vi "Finish.vi"   [LabVIEW 2012]
doc: "This VI is called just before exiting. It is expected to close I/O refnum, save collected data, etc."
uses:
  <vilib>/Rock Robotics/WPI/Compressor/WPI_CompressorGetSetRefNum.vi
  <vilib>/Rock Robotics/WPI/Joystick/WPI_JoystickGetSetRefNum.vi
  <vilib>/Rock Robotics/WPI/RobotDrive/WPI_RobotDriveGetSetRefNum.vi
types:
  T1 = typedef "WPI_MotorControlDeviceRef.ctl" = cluster{"DeviceStatus":errorcluster, "Type":enum16{"PWM", "CAN"}, "PWM":cluster{"Digital Module":T2, "PWM Channel":T3, "DeadBand":T4}, "CAN":cluster{"Device Number":u8, "Control Mode":T5, "Semaphore":T6, "Max Vout":dbl}, "Invert":bool, "TransformRef":T7, "InvTransformRef":T7}
  T2 = typedef "FPGA_TypedefDigitalModule.ctl" = enum16{"Digital Module 1", "Digital Module 2"}
  T3 = typedef "FPGA_DIOPWMChannel.ctl" = enum8{"PWM 1", "PWM 2", "PWM 3", "PWM 4", "PWM 5", "PWM 6", "PWM 7", "PWM 8", "PWM 9", "PWM 10", "Invalid"}
  T4 = typedef "WPI_PWMDeadband.ctl" = cluster{"Name":string, "maxPositivePwm":i32, "minPositivePwm":i32, "centerPwm":i32, "maxNegativePwm":i32, "minNegativePwm":i32, "angularRange":u16}
  T5 = typedef "WPI_CANJaguar_ControlMode.ctl" = enum8{"Percent VBus", "Current", "Speed", "Position", "Voltage"}
  T6 = typedef "Semaphore RefNum" = refnum<k1>
  T7 = typedef "WPI_PWMTransform_ConPane.ctl" = refnum<vi>
  T8 = typedef "WPI_SolenoidDevRef.ctl" = cluster{"DevStatus":errorcluster, "Solenoid Module":T9, "Forward Solenoid Channel":T10, "Reverse Solenoid Channel":T10}
  T9 = typedef "FPGA_TypedefSolenoidModule.ctl" = enum16{"Solenoid Module 1", "Solenoid Module 2"}
  T10 = typedef "WPI_SolenoidChannel.ctl" = enum8{"Solenoid 1", "Solenoid 2", "Solenoid 3", "Solenoid 4", "Solenoid 5", "Solenoid 6", "Solenoid 7", "Solenoid 8", "Invalid"}
  T11 = typedef "WPI_JoystickDevRef.ctl" = cluster{"Device":T12}
  T12 = typedef "WPI_JoystickDeviceEnum.ctl" = enum16{"USB 1", "USB 2", "USB 3", "USB 4", "Kinect 1", "Kinect 2"}
  T13 = typedef "WPI_RelayDevRef.ctl" = cluster{"DevStatus":errorcluster, "Relay Channel":T14, "Digital Module":T2, "Relay Direction":T15}
  T14 = typedef "FPGA_DIORelayChannel.ctl" = enum8{"Relay 1", "Relay 2", "Relay 3", "Relay 4", "Relay 5", "Relay 6", "Relay 7", "Relay 8", "Invalid"}
  T15 = typedef "WPI_RelayDirection.ctl" = enum16{"Both directions", "Forward only", "Reverse only"}
  T16 = typedef "WPI_RobotDriveDevRef.ctl" = cluster{"DevStatus":errorcluster, "Motors[]":T1[], "Square Inputs":bool, "Max Output":dbl, "Isochronous":bool}
  T17 = typedef "WPI_CompressorDevRef.ctl" = cluster{"DevStatus":errorcluster, "DigitalInputDevRef":T18, "RelayDevRef":T13}
  T18 = typedef "WPI_DigitalInputDevRef.ctl" = cluster{"DevStatus":errorcluster, "DIO Channel":T19, "Digital Module":T2}
  T19 = typedef "FPGA_DIOChannel.ctl" = enum8{"DIO 1", "DIO 2", "DIO 3", "DIO 4", "DIO 5", "DIO 6", "DIO 7", "DIO 8", "DIO 9", "DIO 10", "DIO 11", "DIO 12", "DIO 13", "DIO 14", "Invalid"}
  T20 = typedef "WPI_CameraDevRef.ctl" = cluster{"Camera Address":string, "CameraStatus":errorcluster, "Acquire Image Notifier":refnum<notifier>}
  T21 = typedef "WPI_EncoderDevRef.ctl" = cluster{"DevStatus":errorcluster, "EncoderIndex":T22, "CounterIndex":T23, "DistancePerCount":dbl, "Decoding Type":T24}
  T22 = typedef "FPGA_EncoderIdx.ctl" = enum8{"Enc 0", "Enc 1", "Enc 2", "Enc 3", "Invalid"}
  T23 = typedef "FPGA_CounterCtrSystemIndex.ctl" = enum8{"Ctr 0", "Ctr 1", "Ctr 2", "Ctr 3", "Ctr 4", "Ctr 5", "Ctr 6", "Ctr 7", "Invalid"}
  T24 = typedef "WPI_EncoderType.ctl" = enum16{"1x", "2x", "4x"}
  T25 = typedef "WPI_UltrasonicDeviceRef.ctl" = cluster{"DevStatus":errorcluster, "Ping Digital Module":T2, "Echo Digital Module":T2, "Ping Channel":T19, "Echo Channel":T19, "CntIndex":T23}
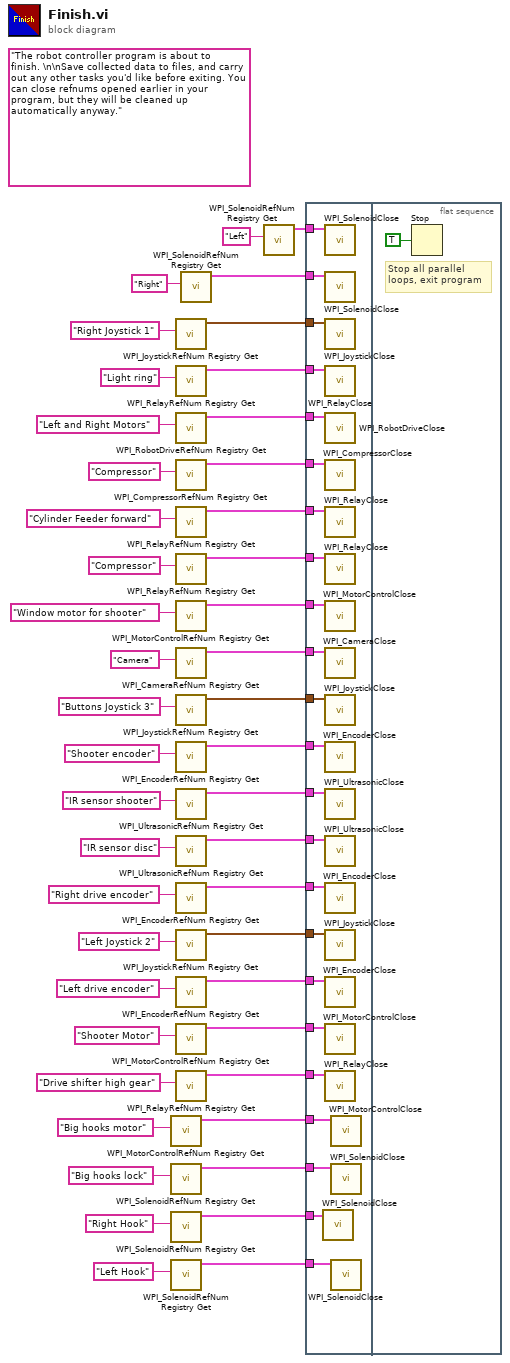
[diagram p0: block diagram]
diagram:
  (unwired) "The robot controller program is about to finish. \n\nSave collected data to files, and carry out any other tasks you'd like before exiting. You can close refnums opened earlier in your program, but they will be cleaned up automatically anyway."
  n1 = call <vilib>:"WPI_MotorControlRefNum Registry Get.vi"("refnum name"="Big hooks motor") -> ("MotorControlDevRef"=w8:T1)  [unwired: 9 in, 1 out]
  n2 = call <vilib>:"WPI_SolenoidRefNum Registry Get.vi"("refnum name"="Big hooks lock") -> ("SolenoidDevRef"=w6:T8)  [unwired: 9 in, 1 out]
  n3 = call <vilib>:"WPI_SolenoidRefNum Registry Get.vi"("refnum name"="Right Hook") -> ("SolenoidDevRef"=w1:T8)  [unwired: 9 in, 1 out]
  n4 = call <vilib>:"WPI_SolenoidRefNum Registry Get.vi"("refnum name"="Left Hook") -> ("SolenoidDevRef"=w2:T8)  [unwired: 9 in, 1 out]
  n5 = call <vilib>:"WPI_JoystickRefNum Registry Get.vi"("refnum name"="Right Joystick 1") -> ("JoystickDevRef"=w43:T11)  [unwired: 1 in, 9 out]
  n6 = call <vilib>:"WPI_RelayRefNum Registry Get.vi"("refnum name"="Light ring") -> ("RelayDevRef"=w9:T13)  [unwired: 9 in, 1 out]
  n7 = call <vilib>:"WPI_RobotDriveRefNum Registry Get.vi"("refnum name"="Left and Right Motors") -> ("RobotDriveDevRef"=w44:T16)  [unwired: 1 in, 9 out]
  n8 = call <vilib>:"WPI_CompressorRefNum Registry Get.vi"("refnum name"="Compressor") -> ("CompressorDevRef"=w20:T17)  [unwired: 9 in, 1 out]
  n9 = call <vilib>:"WPI_RelayRefNum Registry Get.vi"("refnum name"="Cylinder Feeder forward") -> ("RelayDevRef"=w31:T13)  [unwired: 9 in, 1 out]
  n10 = call <vilib>:"WPI_RelayRefNum Registry Get.vi"("refnum name"="Compressor") -> ("RelayDevRef"=w32:T13)  [unwired: 9 in, 1 out]
  n11 = call <vilib>:"WPI_MotorControlRefNum Registry Get.vi"("refnum name"="Window motor for shooter") -> ("MotorControlDevRef"=w13:T1)  [unwired: 9 in, 1 out]
  n12 = call <vilib>:"WPI_CameraRefNum Registry Get.vi"("refnum name"="Camera") -> ("CameraDevRef"=w42:T20)  [unwired: 1 in, 9 out]
  n13 = call <vilib>:"WPI_JoystickRefNum Registry Get.vi"("refnum name"="Buttons Joystick 3") -> ("JoystickDevRef"=w35:T11)  [unwired: 1 in, 9 out]
  n14 = call <vilib>:"WPI_EncoderRefNum Registry Get.vi"("refnum name"="Shooter encoder") -> ("EncoderDevRef"=w11:T21)  [unwired: 9 in, 1 out]
  n15 = call <vilib>:"WPI_UltrasonicRefNum Registry Get.vi"("refnum name"="IR sensor shooter") -> ("UltrasonicDevRef"=w15:T25)  [unwired: 9 in, 1 out]
  n16 = call <vilib>:"WPI_UltrasonicRefNum Registry Get.vi"("refnum name"="IR sensor disc") -> ("UltrasonicDevRef"=w17:T25)  [unwired: 9 in, 1 out]
  n17 = call <vilib>:"WPI_EncoderRefNum Registry Get.vi"("refnum name"="Right drive encoder") -> ("EncoderDevRef"=w25:T21)  [unwired: 9 in, 1 out]
  n18 = call <vilib>:"WPI_JoystickRefNum Registry Get.vi"("refnum name"="Left Joystick 2") -> ("JoystickDevRef"=w37:T11)  [unwired: 1 in, 9 out]
  n19 = call <vilib>:"WPI_EncoderRefNum Registry Get.vi"("refnum name"="Left drive encoder") -> ("EncoderDevRef"=w28:T21)  [unwired: 9 in, 1 out]
  n20 = call <vilib>:"WPI_MotorControlRefNum Registry Get.vi"("refnum name"="Shooter Motor") -> ("MotorControlDevRef"=w39:T1)  [unwired: 9 in, 1 out]
  n21 = call <vilib>:"WPI_RelayRefNum Registry Get.vi"("refnum name"="Drive shifter high gear") -> ("RelayDevRef"=w30:T13)  [unwired: 9 in, 1 out]
  n22 = call <vilib>:"WPI_SolenoidRefNum Registry Get.vi"("refnum name"="Right") -> ("SolenoidDevRef"=w21:T8)  [unwired: 9 in, 1 out]
  n23 = call <vilib>:"WPI_SolenoidRefNum Registry Get.vi"("refnum name"="Left") -> ("SolenoidDevRef"=w23:T8)  [unwired: 9 in, 1 out]
  n24 = flat-sequence {
    tunnel: w44 -> [w69]
    tunnel: w43 -> [w68]
    tunnel: w42 -> [w67]
    tunnel: w39 -> [w66]
    tunnel: w37 -> [w65]
    tunnel: w35 -> [w64]
    tunnel: w32 -> [w63]
    tunnel: w31 -> [w62]
    tunnel: w30 -> [w61]
    tunnel: w28 -> [w60]
    tunnel: w25 -> [w59]
    tunnel: w23 -> [w58]
    tunnel: w21 -> [w57]
    tunnel: w20 -> [w56]
    tunnel: w17 -> [w55]
    tunnel: w15 -> [w54]
    tunnel: w13 -> [w53]
    tunnel: w11 -> [w52]
    tunnel: w9 -> [w51]
    tunnel: w8 -> [w50]
    tunnel: w6 -> [w49]
    tunnel: w2 -> [w48]
    tunnel: w1 -> [w47]
    frame #0 {
      n25 = call <vilib>:"WPI_SolenoidClose.vi"("SolenoidDevRef"=w47) -> ()  [unwired: 10 in, 1 out]
      n26 = call <vilib>:"WPI_SolenoidClose.vi"("SolenoidDevRef"=w58) -> ()  [unwired: 10 in, 1 out]
      n27 = call <vilib>:"WPI_SolenoidClose.vi"("SolenoidDevRef"=w57) -> ()  [unwired: 10 in, 1 out]
      n28 = call <vilib>:"WPI_JoystickClose.vi"("JoystickDevRef"=w68) -> ()  [unwired: 11 out]
      n29 = call <vilib>:"WPI_RelayClose.vi"("RelayDevRef"=w51) -> ()  [unwired: 10 in, 1 out]
      n30 = call <vilib>:"WPI_RobotDriveClose.vi"("RobotDriveDevRef"=w69) -> ()  [unwired: 1 in, 10 out]
      n31 = call <vilib>:"WPI_CompressorClose.vi"("CompressorDevRef"=w56) -> ()  [unwired: 10 in, 1 out]
      n32 = call <vilib>:"WPI_RelayClose.vi"("RelayDevRef"=w62) -> ()  [unwired: 10 in, 1 out]
      n33 = call <vilib>:"WPI_RelayClose.vi"("RelayDevRef"=w63) -> ()  [unwired: 10 in, 1 out]
      n34 = call <vilib>:"WPI_MotorControlClose.vi"("MotorControlDevRef"=w53) -> ()  [unwired: 10 in, 1 out]
      n35 = call <vilib>:"WPI_CameraClose.vi"("CameraDevRef"=w67) -> ()  [unwired: 1 in, 10 out]
      n36 = call <vilib>:"WPI_JoystickClose.vi"("JoystickDevRef"=w64) -> ()  [unwired: 11 out]
      n37 = call <vilib>:"WPI_EncoderClose.vi"("EncoderDevRef"=w52) -> ()  [unwired: 10 in, 1 out]
      n38 = call <vilib>:"WPI_UltrasonicClose.vi"("UltrasonicDevRef"=w54) -> ()  [unwired: 10 in, 1 out]
      n39 = call <vilib>:"WPI_UltrasonicClose.vi"("UltrasonicDevRef"=w55) -> ()  [unwired: 10 in, 1 out]
      n40 = call <vilib>:"WPI_EncoderClose.vi"("EncoderDevRef"=w59) -> ()  [unwired: 10 in, 1 out]
      n41 = call <vilib>:"WPI_JoystickClose.vi"("JoystickDevRef"=w65) -> ()  [unwired: 11 out]
      n42 = call <vilib>:"WPI_EncoderClose.vi"("EncoderDevRef"=w60) -> ()  [unwired: 10 in, 1 out]
      n43 = call <vilib>:"WPI_MotorControlClose.vi"("MotorControlDevRef"=w66) -> ()  [unwired: 10 in, 1 out]
      n44 = call <vilib>:"WPI_RelayClose.vi"("RelayDevRef"=w61) -> ()  [unwired: 10 in, 1 out]
      n45 = call <vilib>:"WPI_MotorControlClose.vi"("MotorControlDevRef"=w50) -> ()  [unwired: 10 in, 1 out]
      n46 = call <vilib>:"WPI_SolenoidClose.vi"("SolenoidDevRef"=w49) -> ()  [unwired: 10 in, 1 out]
      n47 = call <vilib>:"WPI_SolenoidClose.vi"("SolenoidDevRef"=w48) -> ()  [unwired: 10 in, 1 out]
    }
    frame #1 {
      # "Stop all parallel\nloops, exit program"
      n48 = Stop(stop? (T)=TRUE ("Quit")) -> ()
    }
  }
